vi "Initialize.vi"(7 "I2C Channel":u8, 8 "error in (no error)":errorcluster, 10 "Power Mode":T1={"Power Mode and Output Rate"=48, "X-Axis Control"=1, "Y-Axis Control"=2, "Z-Axis Control"=4} {"Z-Axis Control" items=["Z-Axis DISABLE"=0, "Z-Axis ENABLE"=4]; "Y-Axis Control" items=["Y-Axis DISABLE"=0, "Y-Axis ENABLE"=2]; "X-Axis Control" items=["X-Axis DISABLE", "X-Axis ENABLE"]; "Power Mode and Output Rate" items=["Power Down"=0, "Normal Mode @ 50Hz"=32, "Normal Mode @ 100Hz"=40, "Normal Mode @ 400Hz"=48, "Normal Mode @ 1000Hz"=56, "Low-Power @ 0.5Hz"=64, "Low-Power @ 1Hz"=96, "Low-Power @ 2Hz"=128, "Low-Power @ 5Hz"=160, "Low-Power @ 10Hz"=192]}, 11 "LINX Resource In":T2) -> (0 "error out":errorcluster, 3 "LINX Resource Out":T2)   [LabVIEW 2014, in "LMH-LINX.lvlib" / "LIS331HH.lvlib"]
doc: "This VI enables LIS331HH device and puts in Normal Mode @400Hz Output Data Rate (default)\n\n**Author: Stas Legedza"
uses:
  <vilib>/MakerHub/LINX/Public/Sensors/Accelerometer/LIS331HH/LIS331HH.lvlib
  <vilib>/MakerHub/LINX/Private/Type Defs/LINX Ref.ctl
  <vilib>/MakerHub/LINX/Private/Type Defs/Platform.ctl
  <vilib>/MakerHub/LINX/Private/Type Defs/Interface.ctl
  <vilib>/MakerHub/LINX/Private/Device/Type Defs/LINX Device Config.ctl
  <vilib>/MakerHub/LINX/Private/Device/Type Defs/TCP Config.ctl
  <vilib>/MakerHub/LINX/Private/Device/Type Defs/Channels.ctl
  <vilib>/MakerHub/LINX/Public/Sensors/Accelerometer/LIS331HH/_typeDefs/CTRL_REG1.ctl
  <vilib>/MakerHub/LINX/Private/Local IO/LinxI2cWrite.vi
  <vilib>/MakerHub/LINX/Public/Utilities/Check Channel.vi
  <vilib>/MakerHub/LINX/Private/Utilties/Generate Error.vi
  <vilib>/MakerHub/LINX/LMH-LINX.lvlib
  <vilib>/MakerHub/LINX/Private/Device/Device.lvlib
panel:
  # "INPUTS"
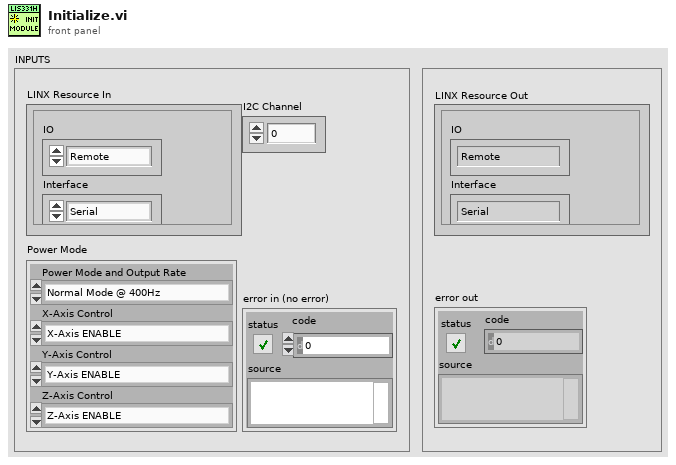
[diagram p1: front panel]
types:
  T1 = typedef "LMH-LINX.lvlib/LIS331HH.lvlib/CTRL_REG1.ctl" = cluster{"Power Mode and Output Rate":u8, "X-Axis Control":u8, "Y-Axis Control":u8, "Z-Axis Control":u8}
  T2 = typedef "LMH-LINX.lvlib/LINX Ref.ctl" = cluster{"IO":T3, "Interface":T4, "LINX Device Config":T5}
  T3 = typedef "LMH-LINX.lvlib/Platform.ctl" = enum16{"Remote", "Local"}
  T4 = typedef "LMH-LINX.lvlib/Interface.ctl" = enum16{"Serial", "TCP"}
  T5 = typedef "LMH-LINX.lvlib/Device.lvlib/LINX Device Config.ctl" = cluster{"Interface":T4, "COM Port":refnum<visa-resource-name>, "TCP Configuration":T6, "Device Family":u8, "Device ID":u8, "Device Name":string, "TCP Ref":refnum<k5>, "Channels":T7}
  T6 = typedef "LMH-LINX.lvlib/Device.lvlib/TCP Config.ctl" = cluster{"IP Address":string, "Port":u16}
  T7 = typedef "LMH-LINX.lvlib/Channels.ctl" = cluster{"DI":u8[], "DO":u8[], "AI":u8[], "AO":u8[], "PWM":u8[], "QE":u8[], "UART":u8[], "I2C 2":u8[], "SPI":u8[], "CAN":u8[], "Servo":u8[], "AI Ref (V)":dbl, "AI Resolution (Bits)":u8, "AO Ref (V)":dbl, "AO Resolution (Bits)":u8}
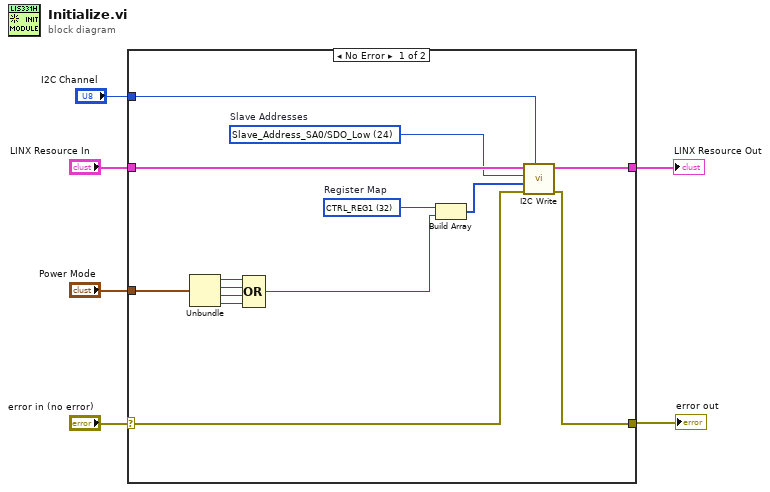
[diagram p0: block diagram]
diagram:
  n1 = case shown="No Error" "error in (no error)" {
    selector: "error in (no error)" -> [w19 w22]
    tunnel: [w15 w22] -> w5
    tunnel: "LINX Resource In" -> [w20 w21]
    tunnel: "I2C Channel" -> [w17 _]
    tunnel: [w16 w21] -> w2
    tunnel: "Power Mode" -> [w12 _]
    frame No Error {
      w13 = u8 24 items=["Slave_Address_SA0/SDO_Low"=24, "Slave_Address_SA0/SDO_High"=25]  # Slave Addresses
      w14 = u8 32 items=["CTRL_REG1"=32, "CTRL_REG2"=33, "CTRL_REG3"=34, "CTRL_REG4"=35, "CTRL_REG5"=36, "HP_FILTER_RESET"=37, "REFERENCE"=38, "STATUS_REG"=39, "OUT_X_L"=40, "OUT_X_H"=41, "OUT_Y_L"=42, "OUT_Y_H"=43, "OUT_Z_L"=44, "OUT_Z_H"=45, "INT1_CFG"=48, "INT1_SOURCE"=49, "INT1_THS"=50, "INT1_DURATION"=51, "INT2_CFG"=52, "INT2_SOURCE"=53, "INT2_THS"=54, "INT2_DURATION"=55]  # Register Map
      n2 = Unbundle(w12) -> ("Power Mode and Output Rate"=w11:u8, "X-Axis Control"=w10:u8, "Y-Axis Control"=w9:u8, "Z-Axis Control"=w8:u8)
      n3 = Compound Arithmetic op=OR(w11, w10, w9, w8) -> (w7:u8)
      n4 = Build Array(w14, w7) -> (w18:u8[])
      n5 = call <vilib>:"I2C Write.vi"("I2C Channel"=w17, "Error In"=w19, "Data"=w18, "I2C Slave Address (0)"=w13, "LINX Resource"=w20) -> ("Error Out"=w15:errorcluster, "LINX Resource"=w16:T2)  [unwired: 5 in]
    }
    frame Error {
    }
  }
  "error out" <- w5
  "LINX Resource Out" <- w2
